vi "Lab17.vi"() -> ()   [LabVIEW 2022 SP3]
uses:
  <vilib>/DAQmx/miscellaneous.llb/DAQmx Fill In Error Info.vi
  <vilib>/DAQmx/configure/trigger.llb/DAQmx Start Trigger (Digital Edge).vi
  <vilib>/DAQmx/create/channels.llb/DAQmx Create Channel (CI-Count Edges).vi
  <vilib>/DAQmx/create/channels.llb/DAQmx Create Channel (CO-Pulse Generation-Time).vi
  <vilib>/DAQmx/read.llb/DAQmx Read (Counter U32 1Chan 1Samp).vi
  <resource>/objmgr/daqmx.rc
panel:
  in  "reset Button":bool
  in  "Trigger":tag
  in  "Count In":tag
  out "Number of Edges":u32
  in  "stop":bool
  in  "Internal Connection":tag="/Dev1/PFI0"
  in  "counter 2":tag="Dev1/ctr1"
  in  "counter":tag="Dev1/ctr0"
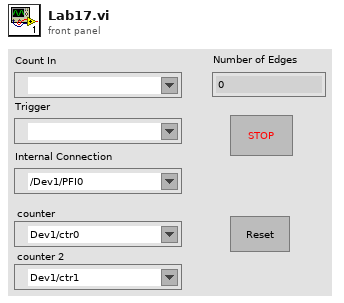
[diagram p1: front panel]
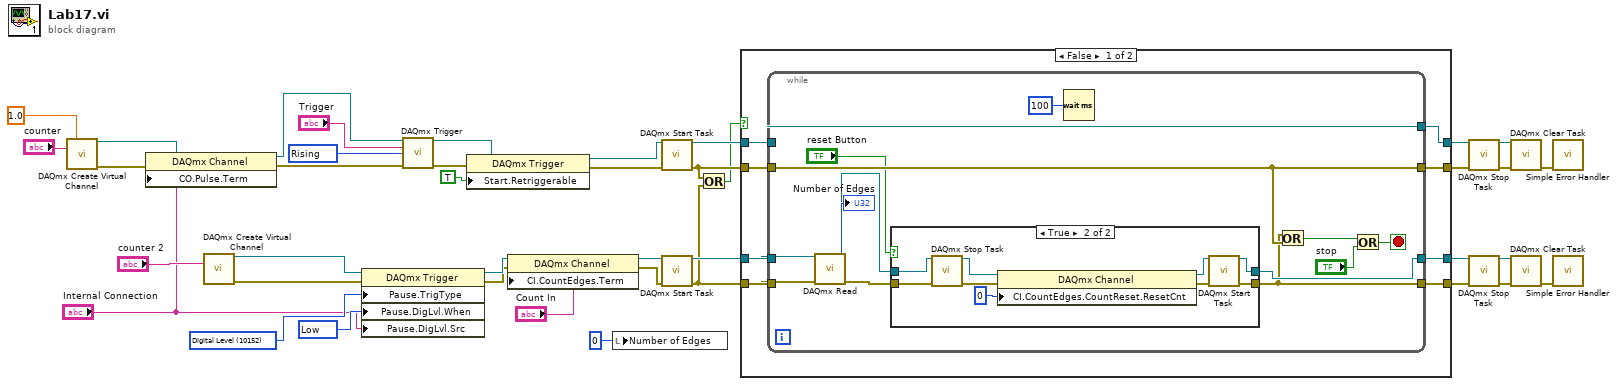
[diagram p0: block diagram]
diagram:
  w33 = 10280 items=["Rising"=10280, "Falling"=10171] ("edge")
  w38 = 10214 items=["High"=10192, "Low"=10214] ("Pause.DigLvl.When")
  w39 = 10152 items=["Analog Level"=10101, "Analog Window"=10103, "Digital Level"=10152, "Digital Pattern"=10398, "None"=10230] ("Pause.TrigType")
  n1 = call-poly <vilib>:"DAQmx Create Virtual Channel.vi"("high time"=1.0, "counter"="counter") -> ("task out"=w28:refnum<k21>, "error out"=w29:errorcluster)  [unwired: 12 in]
  n2 = property class="DAQmx Channel"(reference=w28, error in=w29, "CO.Pulse.Term"="Internal Connection") -> (reference out=w32:refnum<k21>, error out=w31:errorcluster)
  n3 = call-poly <vilib>:"DAQmx Create Virtual Channel.vi"("counter"="counter 2") -> ("task out"=w35:refnum<k21>, "error out"=w34:errorcluster)  [unwired: 13 in]
  n4 = property class="DAQmx Trigger"(reference=w35, error in=w34, "Pause.TrigType"=w39, "Pause.DigLvl.When"=w38, "Pause.DigLvl.Src"="Internal Connection") -> (reference out=w8:refnum<k21>, error out=w5:errorcluster)
  n5 = call-poly <vilib>:"DAQmx Trigger.vi"("task/channels in"=w32, "source"="Trigger", "edge"=w33, "error in"=w31) -> ("task out"=w27:refnum<k21>, "error out"=w26:errorcluster)  [unwired: 10 in]
  n6 = property class="DAQmx Trigger"(reference=w27, error in=w26, "Start.Retriggerable"=TRUE) -> (reference out=w25:refnum<k21>, error out=w24:errorcluster)
  n7 = property class="DAQmx Channel"(reference=w8, error in=w5, "CI.CountEdges.Term"="Count In") -> (reference out=w7:refnum<k21>, error out=w6:errorcluster)
  n8 = local write "Number of Edges"(u32 0 ("Number of Edges")) -> ()
  n9 = call <vilib>:"DAQmx Start Task.vi"("task/channels in"=w25, "error in"=w24) -> ("task out"=w23:refnum<k21>, "error out"=w20:errorcluster)  [unwired: 12 in]
  n10 = call <vilib>:"DAQmx Start Task.vi"("task/channels in"=w7, "error in"=w6) -> ("task out"=w22:refnum<k21>, "error out"=w21:errorcluster)  [unwired: 12 in]
  n11 = Or(x=w20, y=w21) -> (x .or. y?=w19:bool)
  n12 = case shown="False" w19 {
    tunnel: w23 -> [w48 w77]
    tunnel: w22 -> [w46 w75]
    tunnel: w20 -> [w47 w76]
    tunnel: w21 -> [w45 w74]
    tunnel: [w44 w77] -> w17
    tunnel: [w43 w76] -> w18
    tunnel: [w42 w75] -> w10
    tunnel: [w41 w74] -> w9
    frame False {
      n13 = while {
        tunnel: w48 -> [w60]
        tunnel: w46 -> [w62]
        tunnel: w47 -> [w57]
        tunnel: w45 -> [w61]
        tunnel: [w50] -> w42
        tunnel: [w49] -> w41
        tunnel: [w60] -> w44
        tunnel: [w57] -> w43
        stop <- w59 stop-if-true
        n14 = call-poly <vilib>:"DAQmx Read.vi"("task/channels in"=w62, "error in"=w61) -> ("task out"=w52:refnum<k21>, "data"=→"Number of Edges":u32, "error out"=w51:errorcluster)  [unwired: 11 in]
        n15 = case shown="True" "reset Button" {
          tunnel: w52 -> [w64 w72]
          tunnel: w51 -> [w63 w71]
          tunnel: [w64 w67] -> w50
          tunnel: [w63 w65] -> w49
          frame False {
          }
          frame True {
            n16 = call <vilib>:"DAQmx Stop Task.vi"("task/channels in"=w72, "error in"=w71) -> ("task out"=w70:refnum<k21>, "error out"=w69:errorcluster)  [unwired: 12 in]
            n17 = property class="DAQmx Channel"(reference=w70, error in=w69, "CI.CountEdges.CountReset.ResetCnt"=u32 0) -> (reference out=w68:refnum<k21>, error out=w66:errorcluster)
            n18 = call <vilib>:"DAQmx Start Task.vi"("task/channels in"=w68, "error in"=w66) -> ("task out"=w67:refnum<k21>, "error out"=w65:errorcluster)  [unwired: 12 in]
          }
        }
        n19 = Wait (ms)(milliseconds to wait=u32 100) -> ()  [unwired: 1 out]
        n20 = Or(x=w49, y=w57) -> (x .or. y?=w58:bool)
        n21 = Or(x=w58, y="stop") -> (x .or. y?=w59:bool)
      }
    }
    frame True {
    }
  }
  n22 = call <vilib>:"DAQmx Stop Task.vi"("task/channels in"=w17, "error in"=w18) -> ("task out"=w15:refnum<k21>, "error out"=w16:errorcluster)  [unwired: 12 in]
  n23 = call <vilib>:"DAQmx Stop Task.vi"("task/channels in"=w10, "error in"=w9) -> ("task out"=w12:refnum<k21>, "error out"=w13:errorcluster)  [unwired: 12 in]
  n24 = call <vilib>:"DAQmx Clear Task.vi"("task in"=w15, "error in"=w16) -> ("error out"=w14:errorcluster)  [unwired: 13 in]
  n25 = call <vilib>:"DAQmx Clear Task.vi"("task in"=w12, "error in"=w13) -> ("error out"=w11:errorcluster)  [unwired: 13 in]
  n26 = call <vilib>:"Simple Error Handler.vi"("error in (no error)"=w14) -> ()  [unwired: 4 in, 5 out]
  n27 = call <vilib>:"Simple Error Handler.vi"("error in (no error)"=w11) -> ()  [unwired: 4 in, 5 out]
